vi "Test Semaphore 3.vi"() -> ()   [LabVIEW 2011]
panel:
  in  "Handle 2":u16
  out "Iterations":i32
  in  "milliseconds to hold":u32=500
  in  "milliseconds to wait":u32=500
  out "Wait Time":u32
  out "Hold Time":u32
  out "millisecond timer value 1":u32
  out "Prior Count":i32
  out "millisecond timer value 2":u32
  out "Locked 1":bool
  out "Numeric":i32
  out "Timed Out? 1":bool
  out "error out rel 2":errorcluster
  out "error out acq 2":errorcluster
  in  "Acq":bool
  in  "Open":bool
  in  "stop":bool
  out "Handle":u16
  out "error out create":errorcluster
  in  "Name":string="LabVIEW_System_Semaphore"
  out "error out destroy 1":errorcluster
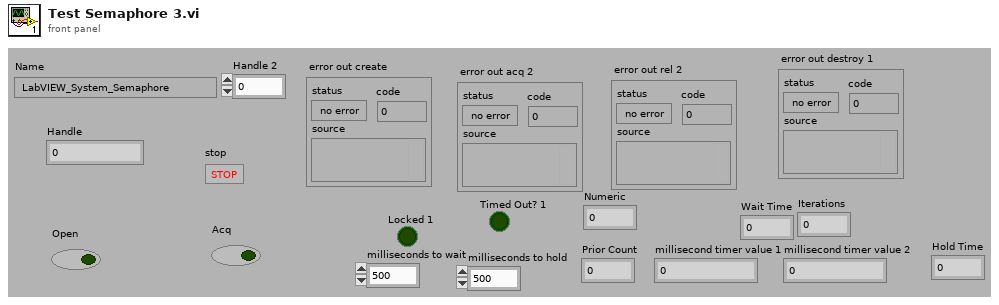
[diagram p1: front panel]
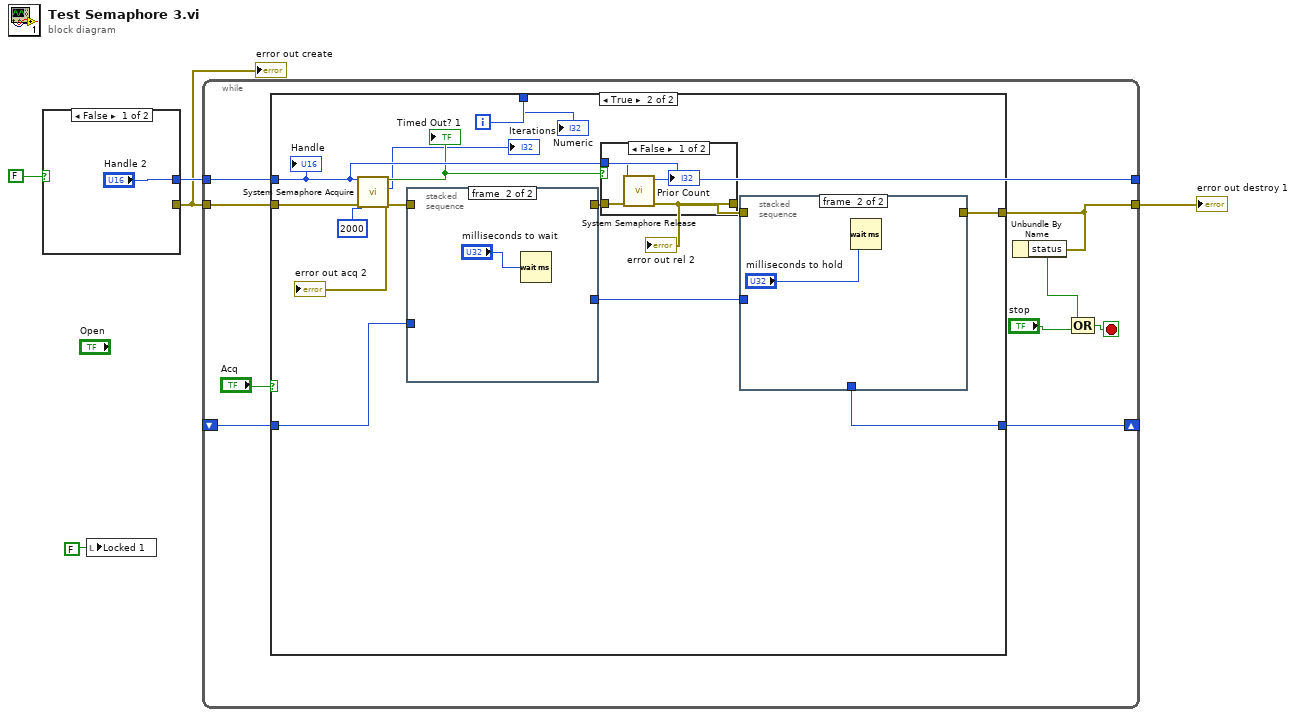
[diagram p0: block diagram]
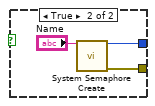
[diagram p2: hidden frame]
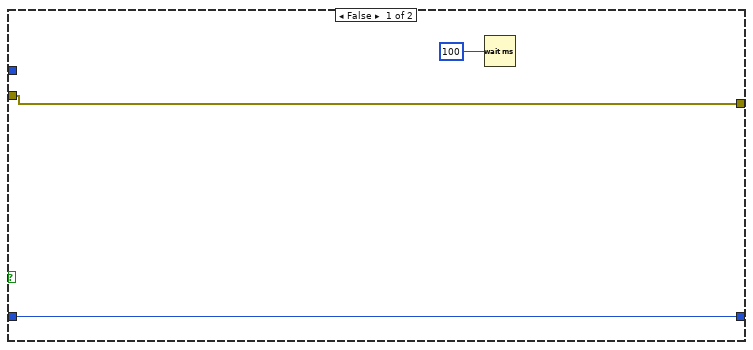
[diagram p3: hidden frame]
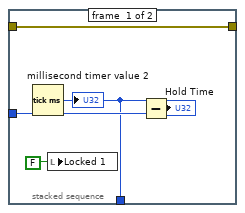
[diagram p5: hidden frame]
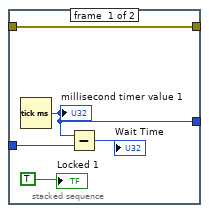
[diagram p6: hidden frame]
diagram:
  n1 = case shown="False" FALSE {
    tunnel: ["Handle 2" w9] -> w5
    tunnel: [_ w8] -> w3
    frame False {
    }
    frame True {
      n2 = call "System Semaphore Create.vi"("Name"="Name") -> ("error out"=w8:errorcluster, "Handle"=w9:u16)  [unwired: 9 in]
    }
  }
  "error out create" <- w3
  n3 = local write "Locked 1"(FALSE) -> ()
  n4 = while {
    tunnel: w3 -> [w12]
    tunnel: w5 -> [w15]
    tunnel: [w15] -> _
    tunnel: [w14] -> w2
    shift-right: [w11] -> _
    shift-left: _ -> [w10]
    i -> [w16]
    stop <- w18 stop-if-true
    n5 = case shown="True" "Acq" {
      tunnel: w16 -> [_ w35]
      tunnel: w15 -> [_ w29]
      tunnel: [w22 w33] -> w14
      tunnel: w12 -> [w22 w28]
      tunnel: [w20 w26] -> w11
      tunnel: w10 -> [w20 w25]
      frame False {
        n6 = Wait (ms)(milliseconds to wait=u32 100) -> ()  [unwired: 1 out]
      }
      frame True {
        n7 = call "System Semaphore Acquire.vi"("error in (no error)"=w28, "Timeout (ms)"=u16 2000, "SemaphoreHandle"=w29) -> ("error out"=w32:errorcluster, "Iterations"=→"Iterations":i16, "Timed Out?"=w24:bool)  [unwired: 6 in]
        "Timed Out? 1" <- w24
        "error out acq 2" <- w32
        n8 = stacked-sequence {
          tunnel: w32 -> [w51 _]
          tunnel: [w51 _] -> w31
          tunnel: [w48 _] -> w27
          tunnel: w25 -> [w47 _]
          frame #0 {
            n9 = Tick Count (ms)() -> (millisecond timer value=w48:u32)
            "millisecond timer value 1" <- w48
            n10 = Subtract(x=w48, y=w47) -> (x-y=→"Wait Time":u32)
            "Locked 1" <- TRUE
          }
          frame #1 {
            n11 = Wait (ms)(milliseconds to wait="milliseconds to wait") -> ()  [unwired: 1 out]
          }
        }
        n12 = case shown="False" w24 {
          tunnel: w31 -> [w39 w40]
          tunnel: w29 -> [w38 _]
          tunnel: [w37 w40] -> w30
          frame False {
            n13 = call "System Semaphore Release.vi"("error in (no error)"=w39, "SemaphoreHandle"=w38) -> ("error out"=w37:errorcluster, "PreviousCount"=→"Prior Count":i32)  [unwired: 8 in]
          }
          frame True {
          }
        }
        "error out rel 2" <- w30
        n14 = stacked-sequence {
          tunnel: w30 -> [w45 _]
          tunnel: [w45 _] -> w33
          tunnel: w27 -> [w43 _]
          tunnel: [w41 _] -> w26
          frame #0 {
            n15 = Tick Count (ms)() -> (millisecond timer value=w41:u32)
            "millisecond timer value 2" <- w41
            n16 = local write "Locked 1"(FALSE) -> ()
            n17 = Subtract(x=w41, y=w43) -> (x-y=→"Hold Time":u32)
          }
          frame #1 {
            n18 = Wait (ms)(milliseconds to wait="milliseconds to hold") -> ()  [unwired: 1 out]
          }
        }
        "Handle" <- w29
        "Numeric" <- w35
      }
    }
    n19 = Unbundle By Name(w14) -> ("status"=w17:bool)
    n20 = Compound Arithmetic op=OR(w17, "stop") -> (w18:bool)
  }
  "error out destroy 1" <- w2
